vi "Control Translator.vi"(11 "JoystickDevRef":T4={"Device"=enum."USB 1"}) -> (1 "D-Pad":T1, 2 "Button Cluster":T2, 3 "Axes":T3)   [LabVIEW 2015]
uses:
  Robot Global Data.vi
  <vilib>/Rock Robotics/WPI/Joystick/WPI_JoystickDeviceEnum.ctl
  <vilib>/Rock Robotics/WPI/Joystick/WPI_JoystickDevRef.ctl
  Common Code/Gamepads/Axes Cluster.ctl
  Common Code/Gamepads/Button Cluster.ctl
  Common Code/Gamepads/D-Pad.ctl
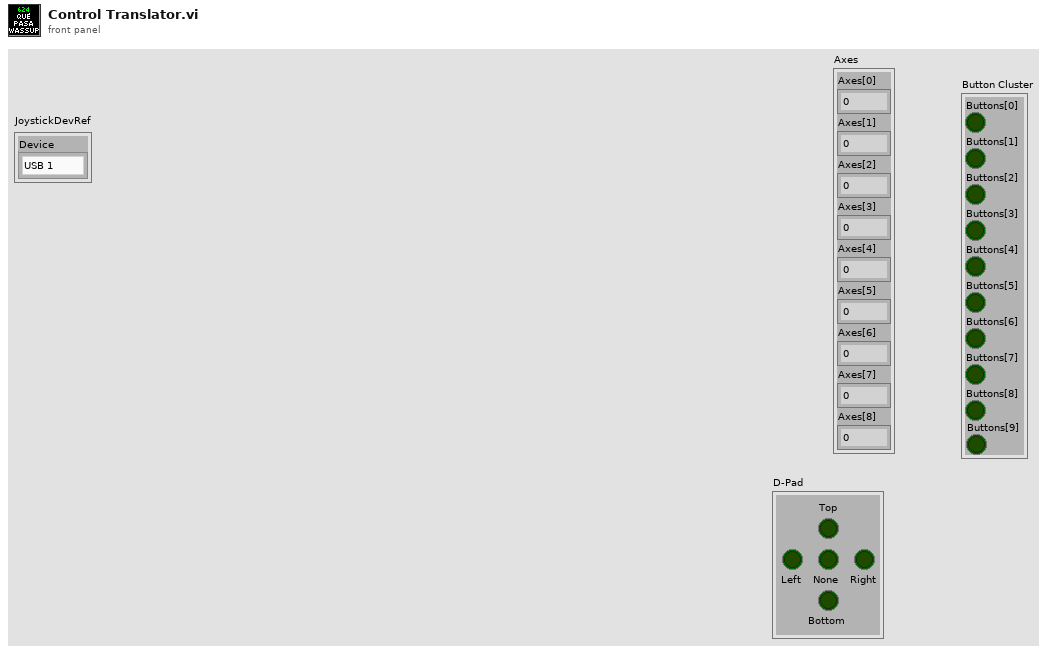
[diagram p1: front panel]
types:
  T1 = typedef "D-Pad.ctl" = cluster{"Top":bool, "Bottom":bool, "None":bool, "Right":bool, "Left":bool}
  T2 = typedef "Button Cluster.ctl" = cluster{"Buttons[0]":bool, "Buttons[1]":bool, "Buttons[2]":bool, "Buttons[3]":bool, "Buttons[4]":bool, "Buttons[5]":bool, "Buttons[6]":bool, "Buttons[7]":bool, "Buttons[8]":bool, "Buttons[9]":bool}
  T3 = typedef "Axes Cluster.ctl" = cluster{"Axes[0]":dbl, "Axes[1]":dbl, "Axes[2]":dbl, "Axes[3]":dbl, "Axes[4]":dbl, "Axes[5]":dbl, "Axes[6]":dbl, "Axes[7]":dbl, "Axes[8]":dbl}
  T4 = typedef "WPI_JoystickDevRef.ctl" = cluster{"Device":T5}
  T5 = typedef "WPI_JoystickDeviceEnum.ctl" = enum16{"USB 0", "USB 1", "USB 2", "USB 3", "USB 4", "USB 5"}
  T6 = typedef "WPI_Joystick Info.ctl" = cluster{"Device Name":string, "HID Type":T7, "XBox Type":T8, "Axes Count":i32, "Axes Types":T9[], "Button Count":i32, "POV Count":i32}
  T7 = typedef "WPI_JoystickHID Types.ctl" = enum16{"Not HID", "HID Joystick", "HID Gamepad", "HID Driving Wheel", "HID Flightstick", "HID First Person"}
  T8 = typedef "WPI_JoystickXBox Types.ctl" = enum16{"Not XBox", "XBox Unknown", "XBox Gamepad", "XBox Wheel", "XBox Arcade Stick", "XBox Flight Stick", "XBox Dance Pad", "XBox Guitar", "XBox Drum Kit", "XBox Arcade Pad"}
  T9 = typedef "WPI_JoystickAxis Types.ctl" = enum16{"X Axis", "Y Axis", "Z Axis", "RxAxis", "RyAxis", "RzAxis", "Slider", "POV", "None", "L X Axis", "L Y Axis", "L Trigger", "R Trigger", "R X Axis", "R Y Axis"}
  T10 = typedef "Manipulator Control Label.ctl" = cluster{"High Pressure Shot":string, "Manual Climb Mode":string, "Auto Climb Mode":string, "Eject":string, "Intake":string, "Manual/Auto Toggle":string, "Re-seat":string, "Intake Down":string}
  T11 = typedef "Driver Control Label.ctl" = cluster{"Outer Shot":string, "Batter Shot":string, "Shoot":string, "Climb":string, "Flashlight":string}
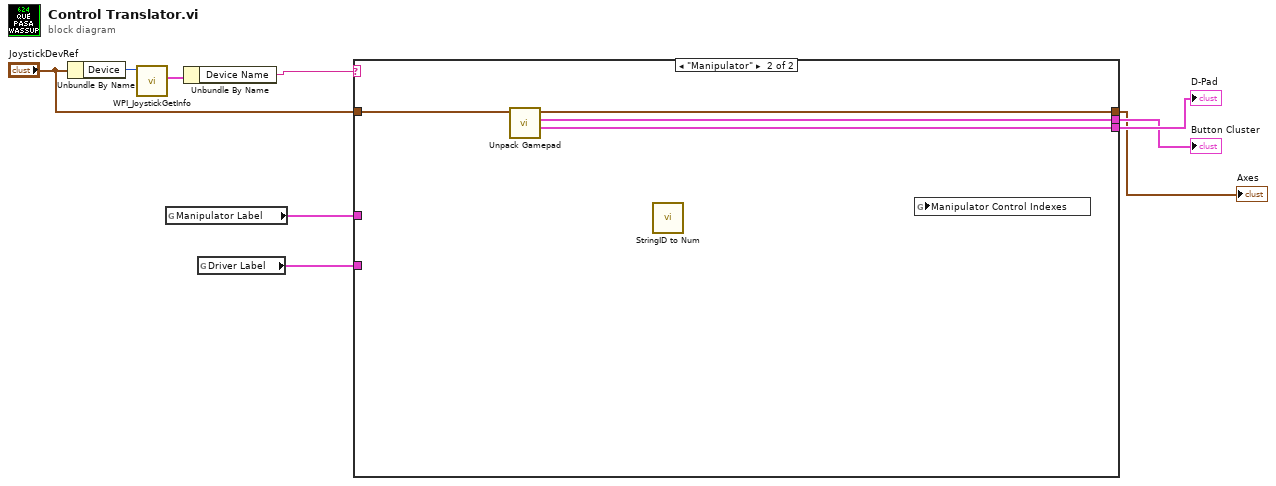
[diagram p0: block diagram]
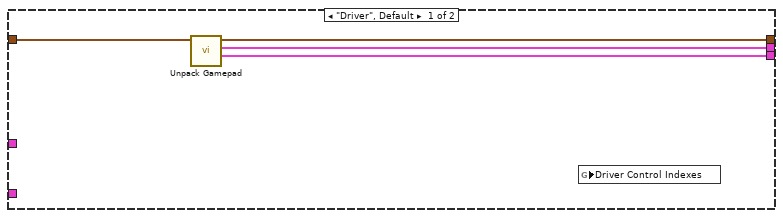
[diagram p2: hidden frame]
diagram:
  n1 = Unbundle By Name("JoystickDevRef") -> ("Device"=w9:T5)
  n2 = call <vilib>:"WPI_JoystickGetInfo.vi"("JoystickDevice"=w9) -> ("Joystick Info"=w8:T6)  [unwired: 9 in, 1 out]
  n3 = global read "Robot Global Data.vi" "Manipulator Label"() -> (w2:T10)
  n4 = Unbundle By Name(w8) -> ("Device Name"=w7:string)
  n5 = global read "Robot Global Data.vi" "Driver Label"() -> (w1:T11)
  n6 = case shown="\"Manipulator\"" w7 {
    tunnel: "JoystickDevRef" -> [w13 w17]
    tunnel: [w12 w16] -> w3
    tunnel: [w11 w15] -> w4
    tunnel: [w10 w14] -> w5
    tunnel: w2 -> [_ _]
    tunnel: w1 -> [_ _]
    frame "Driver", Default {
      n7 = call "Unpack Gamepad.vi"("JoystickDevRef"=w13) -> ("D-Pad"=w10:T1, "Button Cluster"=w11:T2, "Axes"=w12:T3)  [unwired: 8 in]
      n8 = global read "Robot Global Data.vi" "Driver Control Indexes"() -> ()  [unwired: 1 in]
    }
    frame "Manipulator" {
      n9 = call "Unpack Gamepad.vi"("JoystickDevRef"=w17) -> ("D-Pad"=w14:T1, "Button Cluster"=w15:T2, "Axes"=w16:T3)  [unwired: 8 in]
      n10 = call "StringID to Num.vi"() -> ()  [unwired: 11 in, 1 out]
      n11 = global read "Robot Global Data.vi" "Manipulator Control Indexes"() -> ()  [unwired: 1 in]
    }
  }
  "Axes" <- w3
  "Button Cluster" <- w4
  "D-Pad" <- w5
